vi "IrMain.vi"() -> ()   [LabVIEW 2017]
uses:
  <vilib>/addons/InsightCM/Devices/Shared/Common/Trigger/Trigger.lvlib
  <vilib>/addons/TraceLogger/TraceLogger.lvlib
  <vilib>/addons/TimerProcess/TimerProcess.lvlib
  <vilib>/addons/InsightCM/Devices/Shared/Common/Controller/Controller.lvlib
  <vilib>/addons/InsightCM/Devices/Shared/Common/ServerComm/ServerComm.lvlib
  <vilib>/addons/BlinkProcess/BlinkProcess.lvlib
  <vilib>/addons/InsightCM/Devices/Shared/Common/FileManager/FileManager.lvlib
  <vilib>/addons/InsightCM/Devices/Shared/Common/TracePointDisplay/TracePointDisplay.lvlib
  <vilib>/addons/WatchdogProcess/WatchdogProcess.lvlib
  <vilib>/addons/InsightCM/Devices/Shared/Ir/IrAcquisition/IrAcquisition.lvlib
  <vilib>/addons/InsightCM/Devices/Shared/Ir/IrAnalysis/IrAnalysis.lvlib
  <vilib>/addons/InsightCM/Devices/Shared/Ir/IrManageCameras/IrManageCameras.lvlib
  <vilib>/addons/SystemInfoProcess/SystemInfoProcess.lvlib
  <vilib>/addons/InsightCM/Devices/Shared/Common/TrendAlarm/TrendAlarm.lvlib
  <vilib>/addons/InsightCM/Devices/Shared/Ir/IrDataEventCreator/IrDataEventCreator.lvlib
  <vilib>/addons/InsightCM/Utilities/GlobalConfiguration/GlobalConfiguration.lvlib
  <vilib>/addons/InsightCM/Devices/Shared/Ir/IrTestPanel/IrTestPanel.lvlib
  <vilib>/addons/InsightCM/Devices/Shared/Common/DeviceHealth/DeviceHealth.lvlib
  <vilib>/addons/InsightCM/Utilities/PropertyHelpers/PropertyHelpers.lvlib
panel:
  out "debug":string
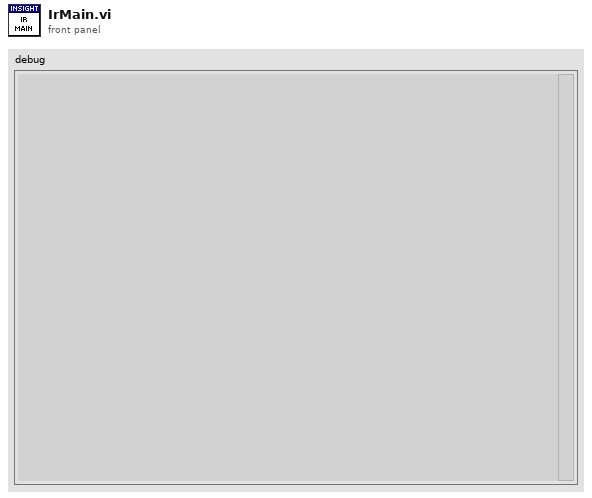
[diagram p1: front panel]
types:
  T1 = typedef "SectionKeyValues.ctl" = cluster{"Section":string, "KeyValues":T2[]}
  T2 = typedef "KeyValuePair.ctl" = cluster{"Key":string, "Value":string}
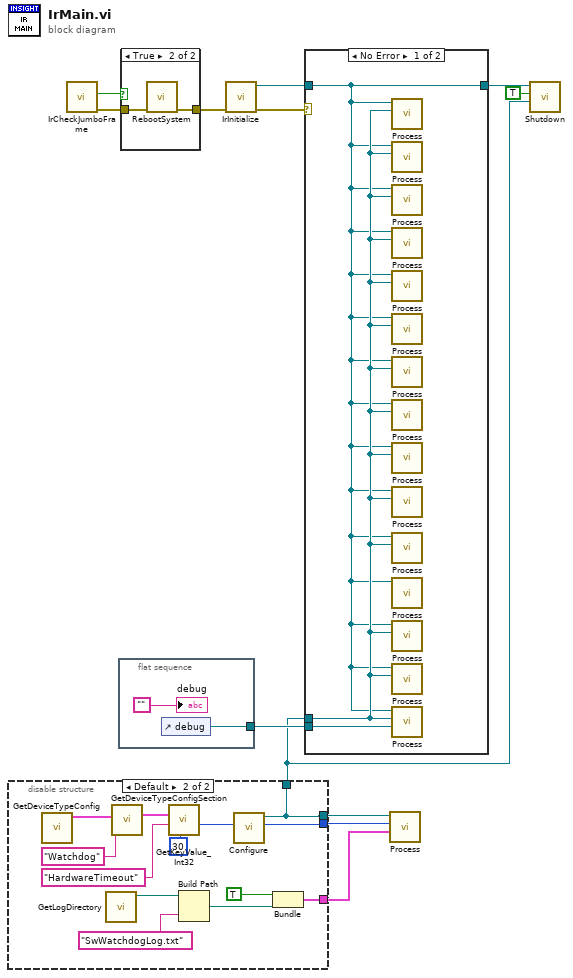
[diagram p0: block diagram]
diagram:
  n1 = disable-structure shown="Default" {
    disable-tunnel: [_ w25] -> w7
    disable-tunnel: [_ w25] -> w9
    disable-tunnel: [_ w24] -> w8
    disable-tunnel: [_ w19] -> w1
    frame condition #0 {
    }
    frame condition #1 (active) {
      n2 = call <vilib>:"GetDeviceTypeConfig.vi"() -> ("key values"=w14:T1[])  [unwired: 9 in, 2 out]
      n3 = call <vilib>:"GetLogDirectory.vi"() -> ("log dir"=w23:path)  [unwired: 10 in, 1 out]
      n4 = call <vilib>:"GetDeviceTypeConfigSection.vi"("key"="Watchdog", "key values"=w14) -> ("key value pairs out"=w17:T2[])  [unwired: 8 in, 1 out]
      n5 = call <vilib>:"GetKeyValue_Int32.vi"("default"=30, "key"="HardwareTimeout" ("Tag"), "key value pairs"=w17) -> ("value"=w13:i32)  [unwired: 6 in, 2 out]
      n6 = Build Path(base path=w23, name or relative path="SwWatchdogLog.txt") -> (appended path=w21:path)
      n7 = call <vilib>:"Configure.vi"("hw timeout (sec)"=w13) -> ("watchdogID out"=w24:u64, "Pound"=w25:refnum<class "Pound.lvclass">)  [unwired: 8 in, 1 out]
      n8 = Bundle(TRUE, "appended path"=w21) -> (w19:cluster{bool, "appended path":path})  [unwired: 1 in]
    }
  }
  n9 = call <vilib>:"IrCheckJumboFrame.vi"() -> ("error out"=w4:errorcluster, "reboot required"=w2:bool)  [unwired: 10 in]
  n10 = flat-sequence {
    tunnel: [w26] -> w11
    frame #0 {
      n11 = control-ref of="debug"() -> (w26:refnum<vi>)
      "debug" <- ""
    }
  }
  n12 = case shown="True" w2 {
    tunnel: w4 -> [w28 w30]
    tunnel: [w28 w29] -> w3
    frame False {
    }
    frame True {
      n13 = call <vilib>:"RebootSystem.vi"("error in (no error)"=w30) -> ("error out"=w29:errorcluster)  [unwired: 10 in]
    }
  }
  n14 = call <vilib>:"IrInitialize.vi"("error in (no error)"=w3) -> ("error out"=w6:errorcluster, "Qbus out"=w5:refnum<class "Qbus.lvclass">)  [unwired: 9 in]
  n15 = case shown="No Error" w6 {
    tunnel: w5 -> [w31 w34]
    tunnel: [w31 w34] -> w12
    tunnel: w7 -> [w32 _]
    tunnel: w11 -> [w33 _]
    frame No Error {
      n16 = call <vilib>:"Process.vi"("Pound in"=w32, "Qbus in"=w31) -> ()  [unwired: 9 in, 1 out]
      n17 = call <vilib>:"Process.vi"("Pound in"=w32, "Qbus in"=w31) -> ()  [unwired: 9 in, 1 out]
      n18 = call <vilib>:"Process.vi"("Pound in"=w32, "Qbus in"=w31) -> ()  [unwired: 9 in, 1 out]
      n19 = call <vilib>:"Process.vi"("Pound in"=w32, "Qbus in"=w31) -> ()  [unwired: 9 in, 1 out]
      n20 = call <vilib>:"Process.vi"("Pound in"=w32, "Qbus in"=w31) -> ()  [unwired: 9 in, 1 out]
      n21 = call <vilib>:"Process.vi"("Pound in"=w32, "Qbus in"=w31) -> ()  [unwired: 9 in, 1 out]
      n22 = call <vilib>:"Process.vi"("Pound in"=w32, "Qbus in"=w31) -> ()  [unwired: 9 in, 1 out]
      n23 = call <vilib>:"Process.vi"("Pound in"=w32, "Qbus in"=w31) -> ()  [unwired: 9 in, 1 out]
      n24 = call <vilib>:"Process.vi"("Pound in"=w32, "Qbus in"=w31) -> ()  [unwired: 9 in, 1 out]
      n25 = call <vilib>:"Process.vi"("Pound in"=w32, "Qbus in"=w31) -> ()  [unwired: 9 in, 1 out]
      n26 = call <vilib>:"Process.vi"("Pound in"=w32, "Qbus in"=w31) -> ()  [unwired: 9 in, 1 out]
      n27 = call <vilib>:"Process.vi"("qbus in"=w31) -> ()  [unwired: 10 in, 1 out]
      n28 = call <vilib>:"Process.vi"("Pound"=w32, "Qbus in"=w31) -> ()  [unwired: 9 in, 1 out]
      n29 = call <vilib>:"Process.vi"("pound in"=w32, "qbus in"=w31) -> ()  [unwired: 9 in, 1 out]
      n30 = call <vilib>:"Process.vi"("string refnum"=w33, "Pound in"=w32, "Qbus in"=w31) -> ()  [unwired: 8 in, 1 out]
    }
    frame Error {
    }
  }
  n31 = call <vilib>:"Process.vi"("Logging"=w1, "watchdogID"=w8, "Pound"=w9) -> ()  [unwired: 6 in, 3 out]
  n32 = call <vilib>:"Shutdown.vi"("Pound"=w7, "restart system"=TRUE, "Qbus in"=w12) -> ()  [unwired: 8 in, 1 out]
